vi "myRIO_BRig_Host_plotCalc_inc.vi"(10 "input_minTrial":i32 caption="input_maxTrialsDisplayed", 11 "input_countTrial":i32) -> (1 "output_min":dbl, 2 "output_max":dbl, 3 "output_inc":dbl)   [LabVIEW 2014]
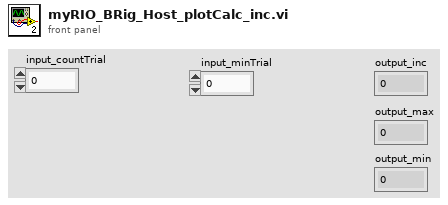
[diagram p1: front panel]
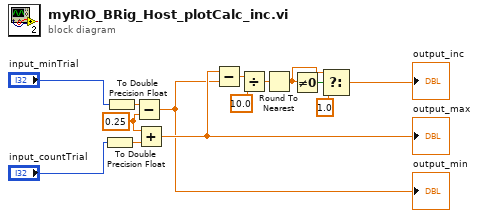
[diagram p0: block diagram]
diagram:
  w12 = 0.25 ("y")
  n1 = To Double Precision Float(number="input_countTrial") -> (double precision float=w13:dbl)
  n2 = To Double Precision Float(number="input_minTrial") -> (double precision float=w14:dbl)
  n3 = Subtract(x=w14, y=w12) -> (x-y=w3:dbl)
  "output_min" <- w3
  n4 = Add(x=w12, y=w13) -> (x+y=w4:dbl)
  "output_max" <- w4
  n5 = Subtract(x=w4, y=w3) -> (x-y=w5:dbl)
  n6 = Divide(x=w5, y=10.0) -> (x/y=w7:dbl)
  n7 = Round To Nearest(number=w7) -> (nearest integer value=w2:dbl)
  n8 = Not Equal To 0?(x=w2) -> (x != 0?=w8:bool)
  n9 = Select(t=w2, s=w8, f=1.0) -> (s? t:f=→"output_inc":dbl)
